vi "read_language_file.vi"(8 "error in":errorcluster, 11 "Text File":path) -> (0 "error out":errorcluster, 3 "gui_strings":string[](array[string]))   [LabVIEW 2013]
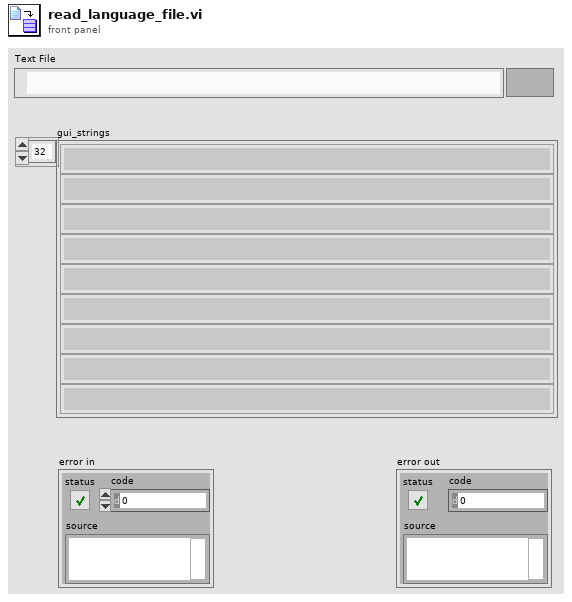
[diagram p1: front panel]
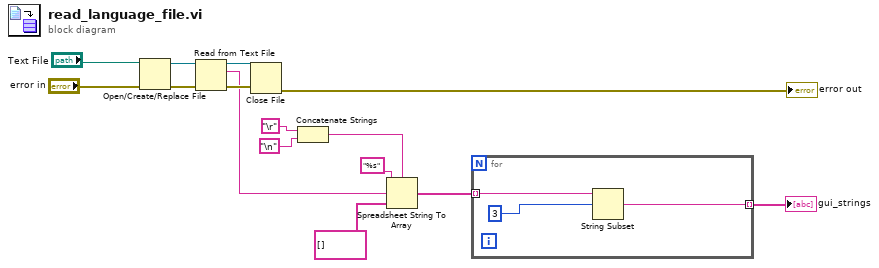
[diagram p0: block diagram]
diagram:
  n1 = Open/Create/Replace File(file path (use dialog)="Text File", error in="error in") -> (refnum out=w13:refnum<file>, error out=w14:errorcluster)  [unwired: 4 in, 1 out]
  n2 = Read from Text File(file (use dialog)=w13, error in=w14) -> (refnum out=w12:refnum<file>, text=w8:string, error out=w11:errorcluster)  [unwired: 2 in, 1 out]
  n3 = Close File(refnum=w12, error in=w11) -> (error out=→"error out":errorcluster)  [unwired: 1 out]
  n4 = Concatenate Strings("\r", "\n") -> (w3:string)
  n5 = Spreadsheet String To Array(delimiter (Tab)=w3, format string="%s", spreadsheet string=w8, array type (2D Dbl)=string[] []) -> (array=w7:string[])
  n6 = for {
    tunnel: w7 -> [w18] mode=indexing
    tunnel: [w16] -> w6 mode=indexing
    n7 = String Subset(string=w18, offset (0)=3) -> (substring=w16:string)  [unwired: 1 in]
  }
  "gui_strings" <- w6
